vi "Write Controller Name.vi"(10 "Controller Name":string, 11 "Timed Loop Controller in":refnum<class "Timed Loop Actor.lvclass">) -> (3 "Timed Loop Controller out":refnum<class "Timed Loop Actor.lvclass">)   [LabVIEW 2025, in "Timed Loop Actor.lvlib" / "Timed Loop Actor.lvclass"]
doc: "This writes the controller name. This name is used just for debugging purposes except on real-time systems, where it is part of the framework for stopping the Timed Loop."
uses:
  Timed Loop Actor.lvclass
  Timed Loop Actor.lvclass/Timed Loop Actor.ctl
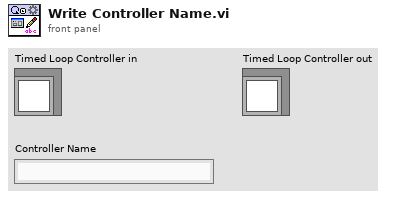
[diagram p1: front panel]
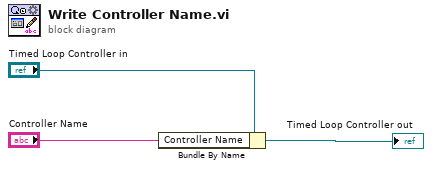
[diagram p0: block diagram]
diagram:
  n1 = Bundle By Name(cluster="Timed Loop Controller in", "Controller Name"="Controller Name") -> (→"Timed Loop Controller out":refnum<class "Timed Loop Actor.lvclass">)
